vi "编辑数据文件.vi"   [LabVIEW 2021]
doc: "本VI是为《我和LabVIEW》一书编写的示例。\n关于本书的介绍请参考网页：\nhttp://ruanqizhen.spaces.live.com/blog/cns!5852D4F797C53FB6!4310.entry"
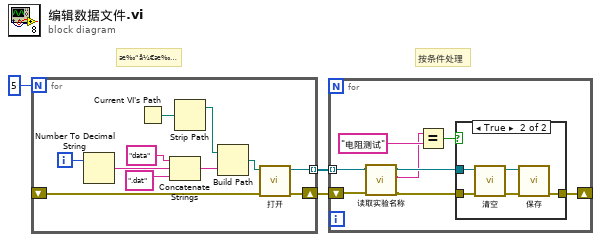
[diagram p0: block diagram]
diagram:
  # "按条件处理"
  # "æ‰“å¼€æ‰€æœ‰æ–‡ä»¶þ"
  n1 = for {
    N: 5 -> [_]
    tunnel: [w4] -> w2 mode=indexing
    shift-right: [w6] -> w1
    shift-left: _ -> [w7]
    i -> [w12]
    n2 = Number To Decimal String(number=w12) -> (decimal integer string=w10:string)  [unwired: 1 out]
    n3 = Current VI's Path() -> (path=w14:path)
    n4 = Concatenate Strings("data" ("名称或相对路径"), w10, ".dat" ("名称或相对路径")) -> (w8:string)
    n5 = Strip Path(path=w14) -> (stripped path=w13:path)  [unwired: 1 out]
    n6 = Build Path(base path=w13, name or relative path=w8) -> (appended path=w5:path)
    n7 = call "打开.vi"("error in (no error)"=w7, "路径"=w5) -> ("error out"=w6:errorcluster, "数据文件.lvclass"=w4:refnum<class "数据文件.lvclass">)  [unwired: 8 in]
  }
  n8 = for {
    tunnel: w2 -> [w19] mode=indexing
    shift-right: [w20] -> _
    shift-left: w1 -> [w18]
    n9 = call-dynamic "读取实验名称.vi"("error in (no error)"=w18, "数据文件.lvclass"=w19) -> ("error out"=w17:errorcluster, "实验名称"=w15:string, "数据文件.lvclass"=w16:refnum<class "数据文件.lvclass">)  [unwired: 7 in]
    n10 = Equal?(x=w15, y="电阻测试") -> (x = y?=w21:bool)
    n11 = case shown="True" w21 {
      tunnel: w16 -> [_ w28]
      tunnel: w17 -> [w23 w27]
      tunnel: [w23 w24] -> w20
      frame False {
      }
      frame True {
        n12 = call-dynamic "清空.vi"("error in (no error)"=w27, "数据文件.lvclass"=w28) -> ("error out"=w25:errorcluster, "数据文件.lvclass"=w26:refnum<class "数据文件.lvclass">)  [unwired: 8 in]
        n13 = call-dynamic "保存.vi"("error in (no error)"=w25, "数据文件.lvclass"=w26) -> ("error out"=w24:errorcluster)  [unwired: 8 in, 1 out]
      }
    }
  }
